vi "MSScript_SubVI_MultipleStr&IndexToSEL.vi"(1 "Expression Sections":cluster{"Str":string, "Start":i32}[](array[cluster])) -> (0 "SEL":cluster{"Start":u32, "End":u32}[](array[cluster]))   [LabVIEW 2018, in "MSScript.lvclass"]
uses:
  MSScript.lvclass
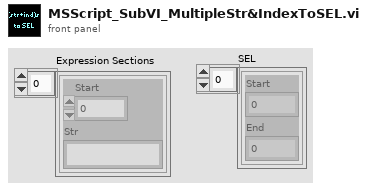
[diagram p1: front panel]
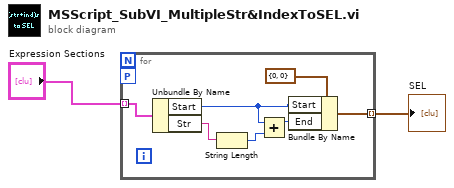
[diagram p0: block diagram]
diagram:
  n1 = for {
    tunnel: "Expression Sections" -> [w4] mode=indexing
    tunnel: [w3] -> w1 mode=indexing
    workers-P: _ -> [_]
    n2 = Unbundle By Name(w4) -> ("Start"=w9:i32, "Str"=w5:string)
    n3 = String Length(string=w5) -> (length=w6:i32)
    n4 = Add(x=w9, y=w6) -> (x+y=w7:i32)
    n5 = Bundle By Name(cluster=cluster{"Start":u32, "End":u32} {"Start"=0, "End"=0}, "Start"=w9, "End"=w7) -> (w3:cluster{"Start":u32, "End":u32})
  }
  "SEL" <- w1
